vi "Get Voltage type.vi"(8 "error in (no error)":errorcluster caption="entrée d'erreur (pas d'erreur)", 11 "Class Multimeter (Default) en entrée":refnum<class "Class Multimeter (Default).lvclass">) -> (0 "error out":errorcluster caption="sortie d'erreur", 2 "Voltage Type":enum16{"AC", "DC"}(ring), 3 "Class Multimeter (Default) en sortie":refnum<class "Class Multimeter (Default).lvclass">)   [LabVIEW 2020, in "Library Instrument & Equipement.lvlib" / "Library Multimeter.lvlib" / "Class Multimeter (Default).lvclass"]
uses:
  Class Multimeter (Default).lvclass
  Class Multimeter (Default).lvclass/Class Multimeter (Default).ctl
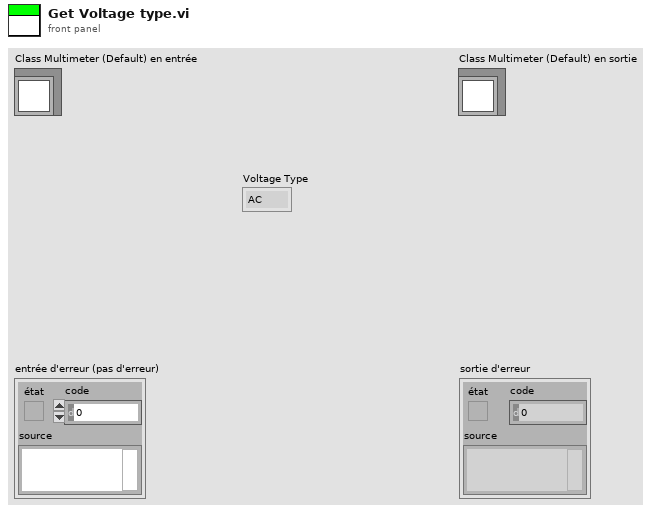
[diagram p1: front panel]
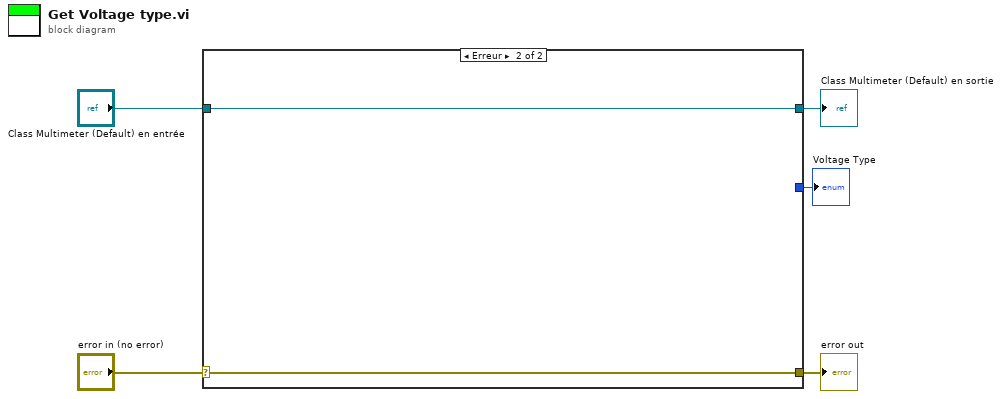
[diagram p0: block diagram]
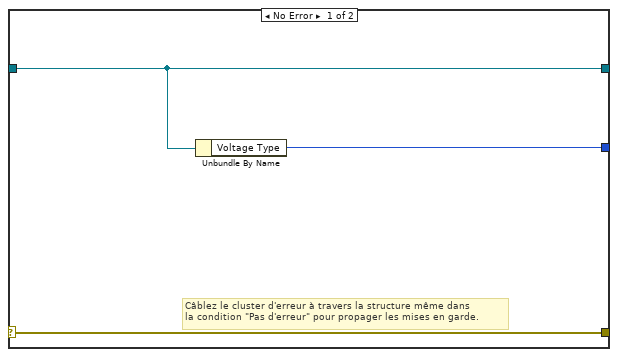
[diagram p2: hidden frame]
diagram:
  n1 = case shown="Erreur" "error in (no error)" {
    selector: "error in (no error)" -> [w8 w10]
    tunnel: [w8 w10] -> w4
    tunnel: [w7 w9] -> w2
    tunnel: "Class Multimeter (Default) en entrée" -> [w7 w9]
    tunnel: [w6 _] -> w1
    frame No Error {
      # "Câblez le cluster d'erreur à travers la structure même dans\nla condition \"Pas d'erreur\" pour propager les mises en garde."
      n2 = Unbundle By Name(w7) -> ("Voltage Type"=w6:enum16{"AC", "DC"})
    }
    frame Error {
    }
  }
  "error out" <- w4
  "Class Multimeter (Default) en sortie" <- w2
  "Voltage Type" <- w1
